vi "Create Header.vi"(0 "task in":refnum<k21>="MyVoltageTask0", 1 "error in":errorcluster) -> (2 "task out":refnum<k21>="MyVoltageTask0", 3 "Array":dbl[](array[numeric]), 4 "error out":errorcluster)   [LabVIEW 2014]
doc: "This VI writes a header to the beginning of the file. It uses the task to get the sample rate and scaling information and saves them as a 1D array of doubles. The exact contents of the array that is saved at the beginning of the file will be the following:\n\nOne double for the number of coefficients in the channel (including sample rate)\nOne double for the number of channels in the task\nAn array of doubles for the device scaling coefficients (including sample rate)"
uses:
  <resource>/objmgr/daqmx.rc
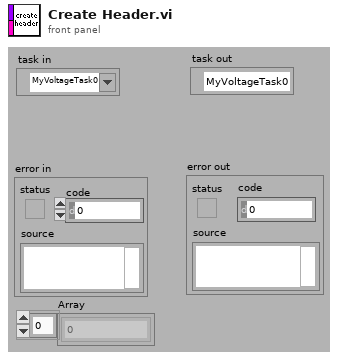
[diagram p1: front panel]
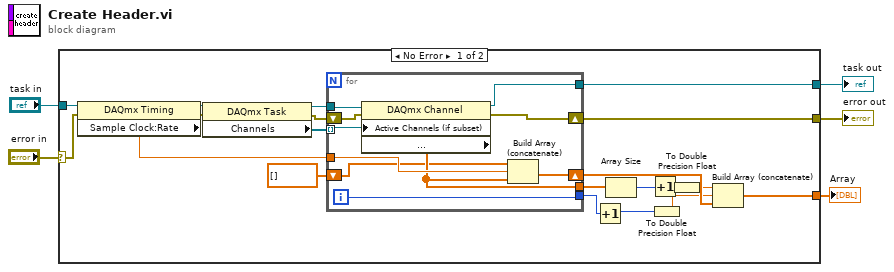
[diagram p0: block diagram]
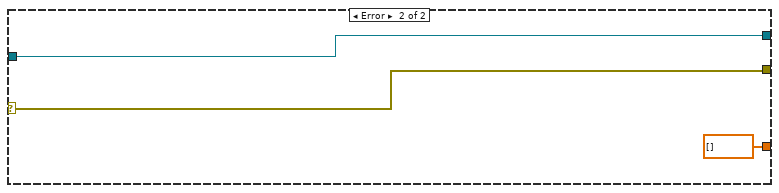
[diagram p2: hidden frame]
diagram:
  n1 = case shown="No Error" "error in" {
    selector: "error in" -> [w17 w37]
    tunnel: "task in" -> [w23 w38]
    tunnel: [w21 w37] -> w4
    tunnel: [w18 w38] -> w3
    tunnel: [w13 dbl[] []] -> w1
    frame No Error {
      n2 = property class="DAQmx Timing"(reference=w23, error in=w17) -> (reference out=w22:refnum<k21>, error out=w20:errorcluster, "Sample Clock:Rate"=w16:dbl)
      n3 = property class="DAQmx Task"(reference=w22, error in=w20) -> (reference out=w19:refnum<k21>, error out=w25:errorcluster, "Channels"=w24:refnum<k21>[])
      n4 = for {
        tunnel: w19 -> [w35]
        tunnel: w24 -> [w33] mode=indexing
        shift-right: [w31] -> w21
        shift-left: w25 -> [w34]
        tunnel: [w32] -> w18
        shift-right: [w30] -> w14
        shift-left: dbl[] [] -> [w26]
        tunnel: w16 -> [w29]
        tunnel: [w28] -> w15
        tunnel: [w27] -> w11
        i -> [w28]
        n5 = property class="DAQmx Channel"(reference=w35, error in=w34, "Active Channels (if subset)"=w33) -> (reference out=w32:refnum<k21>, error out=w31:errorcluster, "Analog Input:General Properties:Advanced:Device Scaling Coefficients:Device Scaling Coefficients"=w27:dbl[])
        n6 = Build Array (concatenate)(w26, w29, w27) -> (w30:dbl[])
      }
      n7 = Increment(x=w15) -> (x+1=w12:i32)
      n8 = Array Size(array=w11) -> (size(s)=w10:i32)
      n9 = Increment(x=w10) -> (x+1=w9:i32)
      n10 = To Double Precision Float(number=w12) -> (double precision float=w7:dbl)
      n11 = To Double Precision Float(number=w9) -> (double precision float=w8:dbl)
      n12 = Build Array (concatenate)(w8, w7, w14) -> (w13:dbl[])
    }
    frame Error {
    }
  }
  "error out" <- w4
  "task out" <- w3
  "Array" <- w1
